vi "语言.vi"(8 "错误输入（无错误）":errorcluster, 9 "背景色":u32(colorbox)=3381759, 11 "Scintilla":refnum<k24>) -> (0 "错误输出":errorcluster, 3 "Scintilla":refnum<k24>)   [LabVIEW 2020]
uses:
  D:/SuperPython-master/ScintillaNET.dll
  ScintillaNET.dll
  D:/SuperPython-master/HightLight.dll
  HightLight.dll
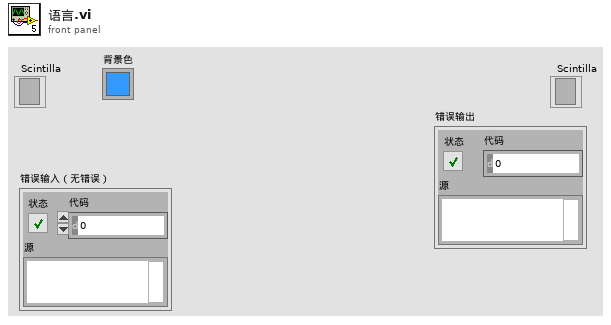
[diagram p1: front panel]
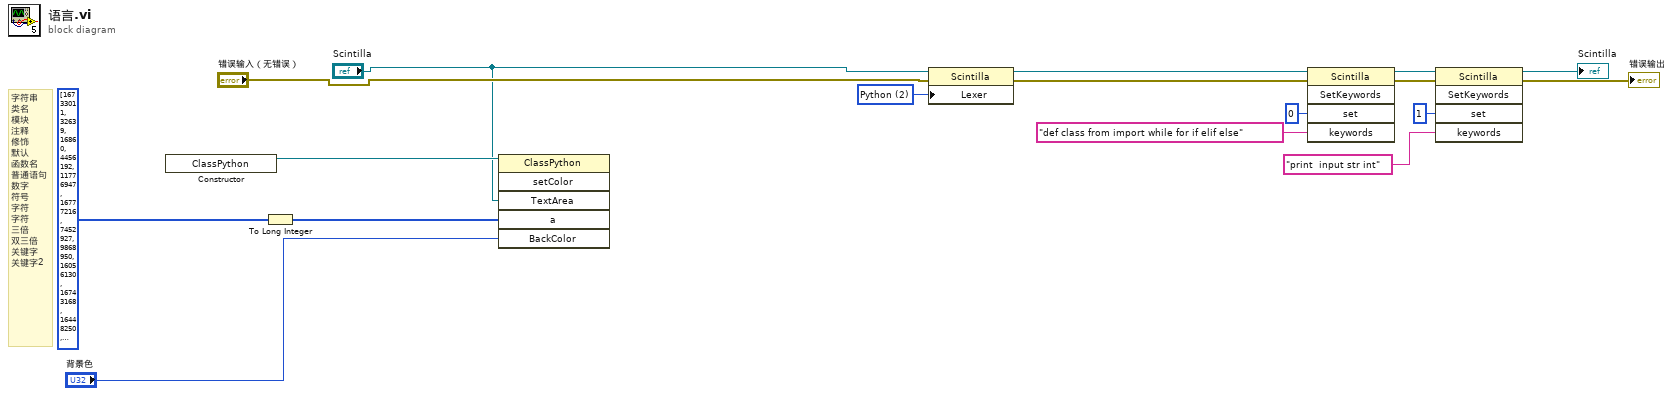
[diagram p0: block diagram]
diagram:
  w13 = 2 items=["Container"=0, "Null"=1, "Python"=2, "Cpp"=3, "Html"=4, "Xml"=5, "Perl"=6, "Sql"=7, "Vb"=8, "Properties"=9, "Batch"=12, "Lua"=15, "Pascal"=18, "Ada"=20, "Lisp"=21, "Ruby"=22, "VbScript"=28, "Asm"=34, "Fortran"=36, "Css"=38, "Verilog"=56, "BlitzBasic"=66, "PureBasic"=67, "PhpScript"=69, "Smalltalk"=72, "FreeBasic"=75, "R"=86, "PowerShell"=88, "Markdown"=98, "Json"=120] ("Lexer")
  # "字符串\n类名\n模块\n注释\n修饰\n默认\n函数名\n普通语句\n数字\n符号\n字符\n字符\n三倍\n双三倍\n关键字\n关键字2"
  n1 = constructor class="ClassPython"() -> (reference out=w12:refnum<k24>)  [unwired: 3 in, 2 out]
  n2 = To Long Integer(number=u32[] [16733011, 32639, 16860, 4456192, 11776947, 16777216, 7452927, 9868950, 16056130, 16743168, 16448250, 16448250, 16448250, 16448250, 16448250, 16448250]) -> (32bit integer=w8:i32[])
  n3 = invoke on="调用节点" class="ClassPython" method="setColor"(reference=w12, "TextArea"="Scintilla", "a"=w8, "BackColor"="背景色") -> ()  [unwired: 2 in, 6 out]
  n4 = property on="属性节点" class="Scintilla"(reference="Scintilla", error in="错误输入（无错误）", "Lexer"=w13) -> (reference out=w15:refnum<k24>, error out=w14:errorcluster)
  n5 = invoke on="调用节点" class="Scintilla" method="SetKeywords"(reference=w15, error in=w14, "set"=0, "keywords"="def class from import while for if elif else") -> (reference out=w4:refnum<k24>, error out=w1:errorcluster)  [unwired: 1 in, 3 out]
  n6 = invoke on="调用节点" class="Scintilla" method="SetKeywords"(reference=w4, error in=w1, "set"=1, "keywords"="print  input str int") -> (reference out=→"Scintilla":refnum<k24>, error out=→"错误输出":errorcluster)  [unwired: 1 in, 3 out]
